vi "Process Updated Vias.vi"(8 "error in (no error)":errorcluster, 10 "Via Paths":path[](array[path]), 11 "GVIWebProcessorApp in":refnum<class "GVIWebProcessorApp.lvclass">) -> (0 "error out":errorcluster, 3 "GVIWebProcessorApp out":refnum<class "GVIWebProcessorApp.lvclass">)   [LabVIEW 2020, in "PicoG-Processor.lvlib" / "GVIWebProcessorApp.lvclass"]
uses:
  GVIWebProcessorApp.lvclass
  Builds/picoG/ppl/PicoG-Core.lvlibp/PicoG-Processor/PicoG-Core/PlatformPluginManager/PlatformPluginManager.lvclass
  Builds/picoG/ppl/PicoG-Core.lvlibp/PicoG-Processor/PicoG-Core/DeployPlatform/DeployPlatform.lvclass
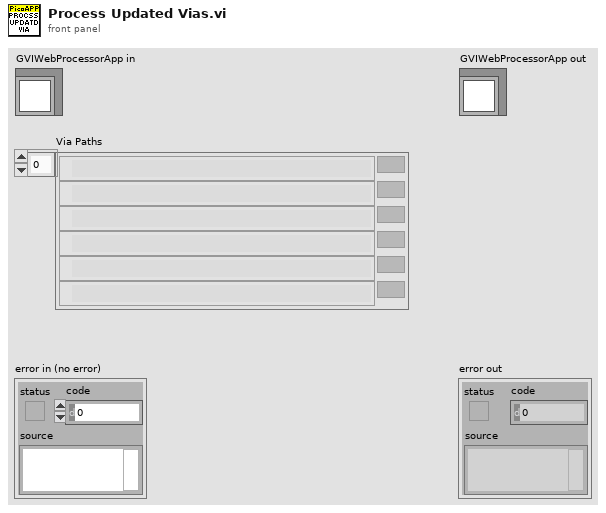
[diagram p1: front panel]
types:
  T1 = typedef "PicoG-Processor.lvlib/GVIWebProcessorApp.lvclass/UI Refs.ctl" = cluster{"Main Window":refnum<vi>, "List Panel":refnum<vi>, "H Splitter":refnum<vi>, "V Splitter":refnum<vi>, "Open Project":refnum<vi>, "Project Name":refnum<vi>, "Auto Process":refnum<vi>, "Auto Deploy":refnum<vi>, "Process Platform":refnum<vi>, "Last Target":refnum<vi>}
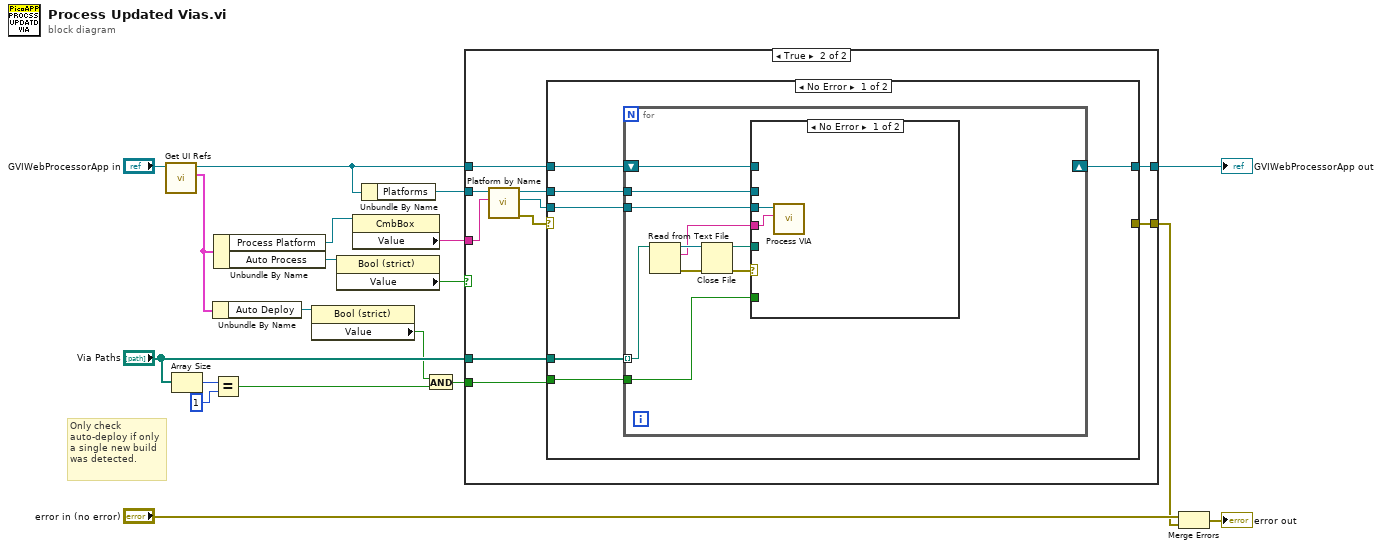
[diagram p0: block diagram]
diagram:
  # "Only check auto-deploy if only a single new build was detected."
  n1 = call "Get UI Refs.vi"("GVIWebProcessorApp in"="GVIWebProcessorApp in") -> ("UI Refs"=w4:T1, "GVIWebProcessorApp out"=w13:refnum<class "GVIWebProcessorApp.lvclass">)  [unwired: 8 in, 1 out]
  n2 = Array Size(array="Via Paths") -> (size(s)=w10:i32)
  n3 = Unbundle By Name(w4) -> ("Auto Deploy"=w3:refnum<vi>)
  n4 = Equal?(x=w10, y=1) -> (x = y?=w8:bool)
  n5 = Unbundle By Name(w4) -> ("Process Platform"=w16:refnum<vi>, "Auto Process"=w17:refnum<vi>)
  n6 = property class="Bool (strict)"(reference=w3) -> ("Value"=w1:bool)  [unwired: 1 in, 2 out]
  n7 = property class="Bool (strict)"(reference=w17) -> ("Value"=w15:bool)  [unwired: 1 in, 2 out]
  n8 = property class="CmbBox"(reference=w16) -> ("Value"=w14:string)  [unwired: 1 in, 2 out]
  n9 = Unbundle By Name(w13) -> ("Platforms"=w12:refnum<class "PlatformPluginManager.lvclass">)
  n10 = And(x=w1, y=w8) -> (x .and. y?=w2:bool)
  n11 = case shown="True" w15 {
    tunnel: w14 -> [_ w29]
    tunnel: w13 -> [w20 w26]
    tunnel: w12 -> [_ w30]
    tunnel: "Via Paths" -> [_ w23]
    tunnel: w2 -> [_ w22]
    tunnel: [w20 w25] -> w7
    tunnel: [_ w24] -> w5
    frame False {
    }
    frame True {
      n12 = call "Platform by Name.vi"("Platform"=w29, "TargetPluginManager in"=w30) -> ("error out"=w28:errorcluster, "Target"=w27:refnum<class "DeployPlatform.lvclass">, "TargetPluginManager out"=w21:refnum<class "PlatformPluginManager.lvclass">)  [unwired: 7 in]
      n13 = case shown="No Error" w28 {
        selector: w28 -> [_ w49]
        tunnel: w27 -> [w36 _]
        tunnel: w26 -> [w34 w50]
        tunnel: [w33 w50] -> w25
        tunnel: [_ w49] -> w24
        tunnel: w23 -> [w35 _]
        tunnel: w22 -> [w32 _]
        tunnel: w21 -> [w31 _]
        frame No Error {
          n14 = for {
            tunnel: w36 -> [w46]
            tunnel: w35 -> [w45] mode=indexing
            shift-right: [_] -> w33
            shift-left: w34 -> [w38]
            tunnel: w32 -> [w40]
            tunnel: w31 -> [w37]
            n15 = Read from Text File(file (use dialog)=w45) -> (refnum out=w43:refnum<file>, text=w41:string, error out=w44:errorcluster)  [unwired: 3 in, 1 out]
            n16 = Close File(refnum=w43, error in=w44) -> (path=w39:path, error out=w42:errorcluster)
            n17 = case shown="No Error" w42 {
              tunnel: w46 -> [w48 _]
              tunnel: w41 -> [w47 _]
              tunnel: w40 -> [_ _]
              tunnel: w39 -> [_ _]
              tunnel: w38 -> [_ _]
              tunnel: w37 -> [_ _]
              frame No Error {
                n18 = call-dynamic "Process VIA.vi"("Raw VIA"=w47, "DeployTarget in"=w48) -> ()  [unwired: 7 in, 3 out]
              }
              frame Error {
              }
            }
          }
        }
        frame Error {
        }
      }
    }
  }
  "GVIWebProcessorApp out" <- w7
  n19 = Merge Errors("error in (no error)", w5) -> (→"error out":errorcluster)
